vi "main.vi"(8 "error in":errorcluster) -> (0 "error out":errorcluster)   [LabVIEW 2018, in "Entry Console.lvlib"]
uses:
  Entry Console.lvlib
  Common/Common.lvlib
  Common/vi/Stop All - Action.ctl
  ctl/Queue Actions.ctl
  ctl/Module State.ctl
  Error Handler/Error Handler/ctl/Module State.ctl
  Error Handler/Error Handler/Error Handler.lvlib
  Controller/Controller.lvlib
  Controller/ctl/Module State.ctl
  ctl/Wash Step Selection Buttons.ctl
panel:
  in  "Start":bool
  in  "Wash Step Selection Buttons":T1
  # "Entry Console"
  # "[Covers: UI1]"
  # "[Covers: UI2]"
  # "[Covers: UI2A]\n[Covers: UI2A1]"
  # "[Covers: UI2A2]"
  # "See mechanical action"
  # "[Covers: UI2B]"
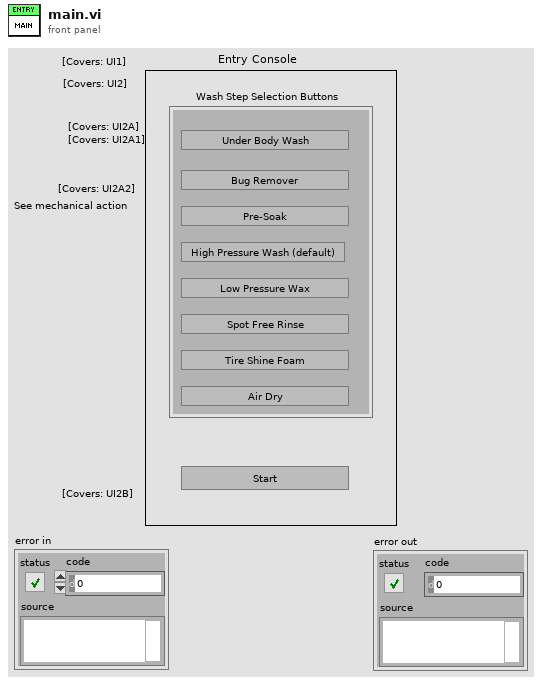
[diagram p1: front panel]
types:
  T1 = typedef "Entry Console.lvlib/Wash Step Selection Buttons.ctl" = cluster{"Under Body Wash":bool, "Bug Remover":bool, "Pre-Soak":bool, "High Pressure Wash (default)":bool, "Low Pressure Wax":bool, "Spot Free Rinse":bool, "Tire Shine Foam":bool, "Air Dry":bool}
  T2 = typedef "Entry Console.lvlib/Module State.ctl" = enum16{"Init", "Idle", "Error", "Close", "Wash Step Selection Buttons: Enable/Disable All", "Wash Step Selection Buttons: Set All", "Wash Step Selection Buttons: Set Single (On/Off)", "Start: Enable/Disable", "Start: Set State (On/Off)"}
  T3 = typedef "Entry Console.lvlib/Queue Actions.ctl" = enum16{"Create", "Get", "Destroy"}
  T4 = typedef "Common.lvlib/Stop All - Action.ctl" = enum16{"Create", "Get", "Fire", "Destroy"}
  T5 = typedef "Controller.lvlib/Module State.ctl" = enum16{"Init", "Idle", "Error", "Close", "Wait for Start State", "Start State", "Wait For Vehicle Position", "Wash Step Execution", "Wash Step/Cycle Completion", "Wash Exit State", "Wash Abort/Terminate State", "Entry Console: Start button pressed", "Entry Console: Wash Steps buttons Pressed", "Vehicle Position: Slider Moved", "Check Timer"}
  T6 = typedef "Error Handler.lvlib/Module State.ctl" = enum16{"Init", "Idle", "Error", "Close", "Handle External Error", "Log Error"}
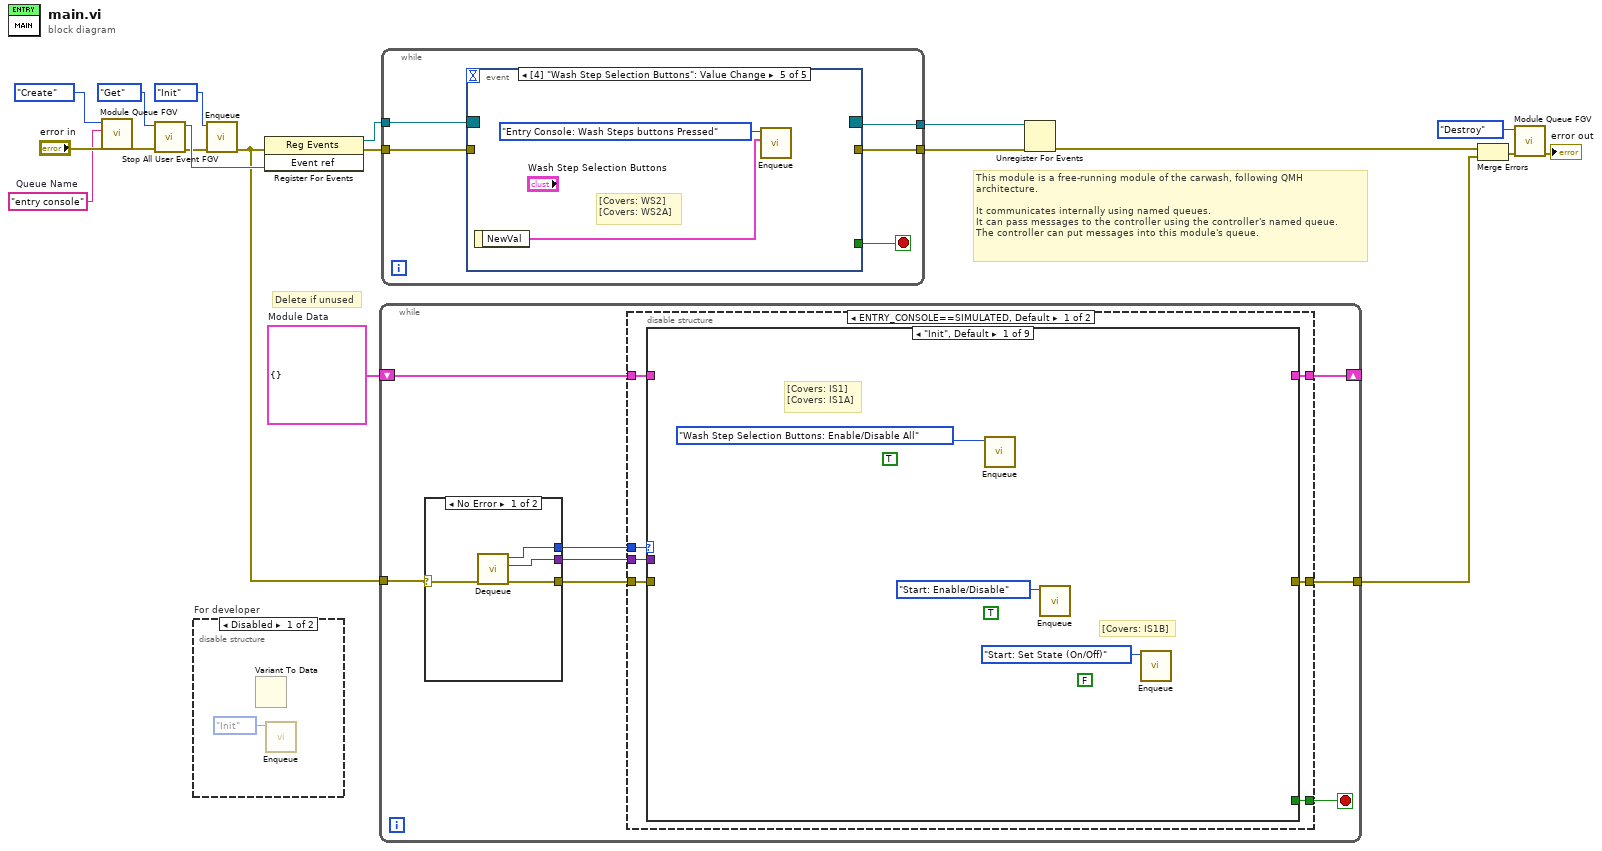
[diagram p0: block diagram]
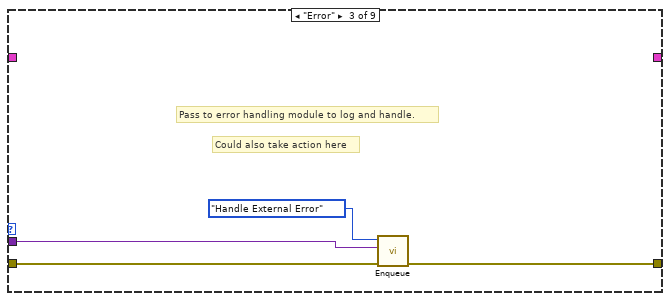
[diagram p4: hidden frame]
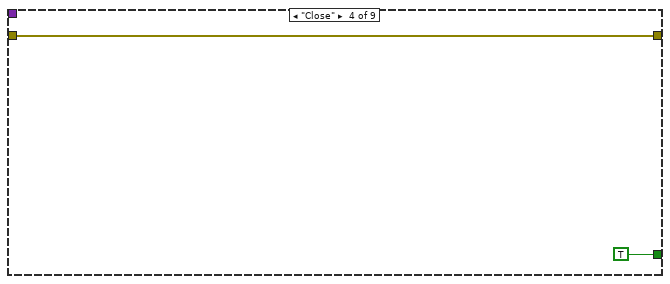
[diagram p5: hidden frame]
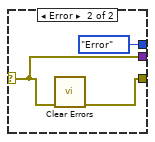
[diagram p12: hidden frame]
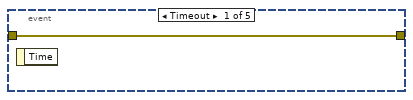
[diagram p13: hidden frame]
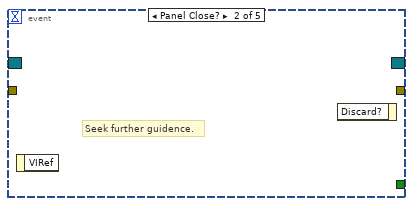
[diagram p14: hidden frame]
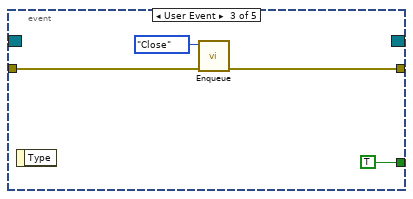
[diagram p15: hidden frame]
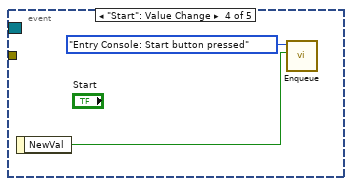
[diagram p16: hidden frame]
diagram:
  w1 = "entry console"  # Queue Name
  w6 = cluster{} {}  # Module Data
  # "This module is a free-running module of the carwash, following QMH\narchitecture.\n\nIt communicates internally using named queues.\nIt can pass messages to the controller using the controller's named queue.\nThe controller can put messages into this module's queue."
  # "Delete if unused"
  n1 = call "Module Queue FGV.vi"("error in"="error in", "Queue Name"=w1, "Action"=Queue_Actions."Create") -> ("error out"=w16:errorcluster)  [unwired: 7 in, 1 out]
  n2 = call "Stop All User Event FGV.vi"("error in"=w16, "Action"=Stop_All_-_Action."Get") -> ("error out"=w15:errorcluster, "Event ref"=w18:refnum<user-event>)  [unwired: 8 in]
  n3 = disable-structure "For developer" shown="Disabled" {
    frame Disabled {
      n4 = Variant To Data() -> ()  [unwired: 3 in, 2 out]
      n5 = call "Enqueue.vi"("State"=Module_State."Init") -> ()  [unwired: 10 in, 1 out]
    }
    frame Enabled {
    }
  }
  n6 = call "Enqueue.vi"("error in"=w15, "State"=Module_State."Init") -> ("error out"=w7:errorcluster)  [unwired: 9 in]
  n7 = register-events(error in=w7, w18) -> (reference out=w13:refnum<event-registration>, error out=w11:errorcluster)  [unwired: 1 in]
  n8 = while {
    tunnel: w7 -> [w28]
    shift-right: [w23] -> _
    shift-left: w6 -> [w24]
    tunnel: [w21] -> w5
    stop <- w22 stop-if-true
    n9 = case shown="No Error" w28 {
      selector: w28 -> [w49 w51]
      tunnel: [w48 w52] -> w25
      tunnel: [w47 w51] -> w26
      tunnel: [w46 Module_State."Error" ("State")] -> w27
      frame No Error {
        n10 = call "Dequeue.vi"("error in"=w49) -> ("error out"=w48:errorcluster, "Data"=w47:variant, "State"=w46:T2)  [unwired: 8 in]
      }
      frame Error {
        n11 = call <vilib>:"Clear Errors.vi"("error in (no error)"=w51) -> ("error out"=w52:errorcluster)  [unwired: 5 in, 1 out]
      }
    }
    n12 = disable-structure shown="ENTRY_CONSOLE==SIMULATED, Default" {
      disable-tunnel: w27 -> [w35 _]
      disable-tunnel: w26 -> [w34 _]
      disable-tunnel: w25 -> [w33 _]
      disable-tunnel: w24 -> [w32 _]
      disable-tunnel: [w31 _] -> w23
      disable-tunnel: [w30 _] -> w22
      disable-tunnel: [w29 _] -> w21
      frame condition #0 (active) {
        n13 = case shown="\"Init\", Default" w35 {
          tunnel: w34 -> [_ _ w41 _ _ _ _ _ _]
          tunnel: w33 -> [_ _ w40 w44 _ _ _ _ _]
          tunnel: w32 -> [_ w39 _ _ _ _ _ _ _]
          tunnel: [_ w39 _ _ _ _ _ _ _] -> w31
          tunnel: [_ _ _ TRUE _ _ _ _ _] -> w30
          tunnel: [_ _ w42 w44 _ _ _ _ _] -> w29
          frame "Init", Default {
            (unwired) FALSE
            (unwired) TRUE
            (unwired) TRUE
            # "[Covers: IS1B]"
            # "[Covers: IS1]\n[Covers: IS1A]"
            n14 = call "Enqueue.vi"("State"=Module_State."Wash Step Selection Buttons: Enable/Disable All") -> ()  [unwired: 10 in, 1 out]
            n15 = call "Enqueue.vi"("State"=Module_State."Start: Enable/Disable") -> ()  [unwired: 10 in, 1 out]
            n16 = call "Enqueue.vi"("State"=Module_State."Start: Set State (On/Off)") -> ()  [unwired: 10 in, 1 out]
          }
          frame "Idle" {
          }
          frame "Error" {
            # "Could also take action here"
            # "Pass to error handling module to log and handle."
            n17 = call "Enqueue.vi"("error in"=w40, "Data"=w41, "State"=Module_State."Handle External Error") -> ("error out"=w42:errorcluster)  [unwired: 8 in]
          }
          frame "Close" {
          }
          frame "Wash Step Selection Buttons: Enable/Disable All" {
          }
          frame "Wash Step Selection Buttons: Set All" {
          }
          frame "Wash Step Selection Buttons: Set Single (On/Off)" {
          }
          frame "Start: Enable/Disable" {
          }
          frame "Start: Set State (On/Off)" {
          }
        }
      }
      frame condition #1 {
        # "Insert hardware code here - see other case"
      }
    }
  }
  n18 = while {
    tunnel: w13 -> [w57]
    tunnel: [w56] -> w12
    tunnel: [w55] -> w10
    tunnel: w11 -> [w54]
    stop <- w53 stop-if-true
    n19 = event shown="[4] \"Wash Step Selection Buttons\": Value Change" {
      selector: w57 -> [_ _ _ _ _]
      dyn-events: [_ _ _ _ _] -> w56
      timeout: _ -> [_ _ _ _ _]
      tunnel: [w58 _ w61 _ _] -> w55
      tunnel: w54 -> [w58 _ w62 _ _]
      tunnel: [_ _ TRUE _ _] -> w53
      event Timeout {
        n20 = event-data() -> ()  [unwired: 1 in, 1 out]
      }
      event Panel Close? {
        # "Seek further guidence."
        n21 = event-data() -> ()  [unwired: 1 in, 1 out]
        n22 = event-data() -> ()  [unwired: 2 in, 1 out]
      }
      event User Event {
        n23 = event-data() -> ()  [unwired: 1 in, 1 out]
        n24 = call "Enqueue.vi"("error in"=w62, "State"=Module_State."Close") -> ("error out"=w61:errorcluster)  [unwired: 9 in]
      }
      event "Start": Value Change {
        n25 = event-data() -> ("NewVal"=w63:bool)  [unwired: 1 in]
        n26 = call "Enqueue.vi"("Data"=w63, "State"=Module_State."Entry Console: Start button pressed") -> ()  [unwired: 9 in, 1 out]
      }
      event Value Change {
        # "[Covers: WS2]\n[Covers: WS2A]"
        n27 = event-data() -> ("NewVal"=w65:T1)  [unwired: 1 in]
        n28 = call "Enqueue.vi"("Data"=w65, "State"=Module_State."Entry Console: Wash Steps buttons Pressed") -> ()  [unwired: 9 in, 1 out]
      }
    }
  }
  n29 = Unregister For Events(event registration refnum=w12, error in=w10) -> (error out=w2:errorcluster)
  n30 = Merge Errors(w2, w5) -> (w4:errorcluster)
  n31 = call "Module Queue FGV.vi"("error in"=w4, "Action"=Queue_Actions."Destroy") -> ("error out"=→"error out":errorcluster)  [unwired: 8 in, 1 out]
